vi "HEWH Heat Elements Interpretation.vi"(0 "POWER":T1) -> (4 "Heat or Fan No Error":bool, 6 "UE and No Error":bool, 8 "Com and No Error":bool, 10 "Comp or HE No Error":bool)   [LabVIEW 2014]
uses:
  Type Definitions/PowerElements.ctl
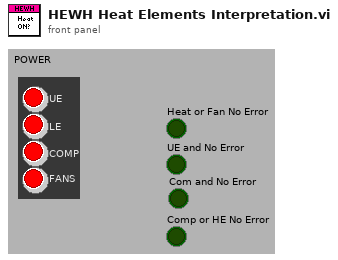
[diagram p1: front panel]
types:
  T1 = typedef "PowerElements.ctl" = cluster{"UE":bool, "LE":bool, "COMP":bool, "FANS":bool}
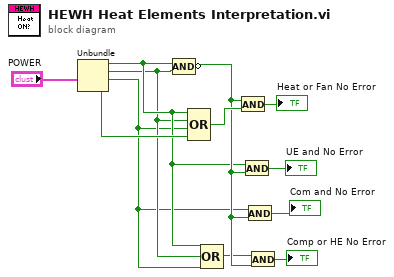
[diagram p0: block diagram]
diagram:
  n1 = Unbundle("POWER") -> ("UE"=w3:bool, "LE"=w2:bool, "COMP"=w1:bool, "FANS"=w11:bool)
  n2 = Compound Arithmetic op=AND(w3, w2) -> (invert w6:bool)
  n3 = Compound Arithmetic op=OR(w3, w2, w1, w11) -> (w9:bool)
  n4 = Compound Arithmetic op=OR(w3, w2, w1) -> (w4:bool)
  n5 = And(x=w6, y=w9) -> (x .and. y?=→"Heat or Fan No Error":bool)
  n6 = And(x=w3, y=w6) -> (x .and. y?=→"UE and No Error":bool)
  n7 = And(x=w1, y=w6) -> (x .and. y?=→"Com and No Error":bool)
  n8 = And(x=w4, y=w6) -> (x .and. y?=→"Comp or HE No Error":bool)
